vi "Initalise TX Queue Ref.vi"(8 "Error In":errorcluster) -> (0 "error out":errorcluster, 3 "TX Queue Out":refnum<queue>)   [LabVIEW 2014]
uses:
  Aircraft Information/Sub VI/Selected Aircraft/SubVI/Get Selected Aircraft.vi
  Aircraft Data Router/SubVI/Queue References/SubVI/Get Aircraft TX Queue String.vi
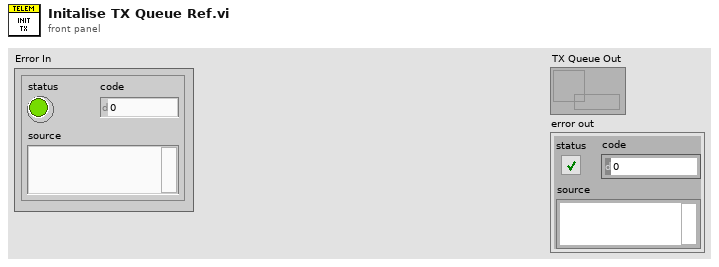
[diagram p1: front panel]
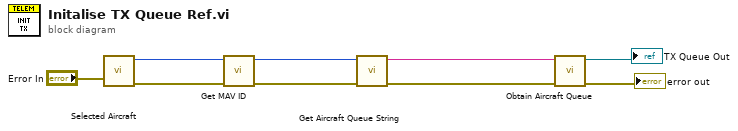
[diagram p0: block diagram]
diagram:
  n1 = call-poly "Selected Aircraft.vi"("Error In"="Error In") -> ("Error Out"=w2:errorcluster, "Selected Aircraft ID Out"=w3:u8)  [unwired: 9 in]
  n2 = call "Get MAV ID.vi"("Error In"=w2, "Aircraft Index"=w3) -> ("Error Out"=w7:errorcluster, "Aircraft ID"=w8:u8)  [unwired: 8 in]
  n3 = call-poly "Get Aircraft Queue String.vi"("Error In"=w7, "Aircraft ID"=w8) -> ("Error Out"=w6:errorcluster, "Aircraft Queue Name"=w9:string)  [unwired: 8 in]
  n4 = call "Obtain Aircraft Queue.vi"("error in (no error)"=w6, "Queue Name"=w9) -> ("error out"=→"error out":errorcluster, "queue out"=→"TX Queue Out":refnum<queue>)  [unwired: 8 in]
